vi "Manual Mode Update Vacuum.vi"(8 "error in":errorcluster, 10 "Vacuum Status":T1, 11 "Gantry in":refnum<class "Gantry Class.lvclass">) -> (0 "error out":errorcluster, 3 "Gantry out":refnum<class "Gantry Class.lvclass">)   [LabVIEW 2011]
uses:
  Shared Components/Gantry Class/Gantry Class.lvclass
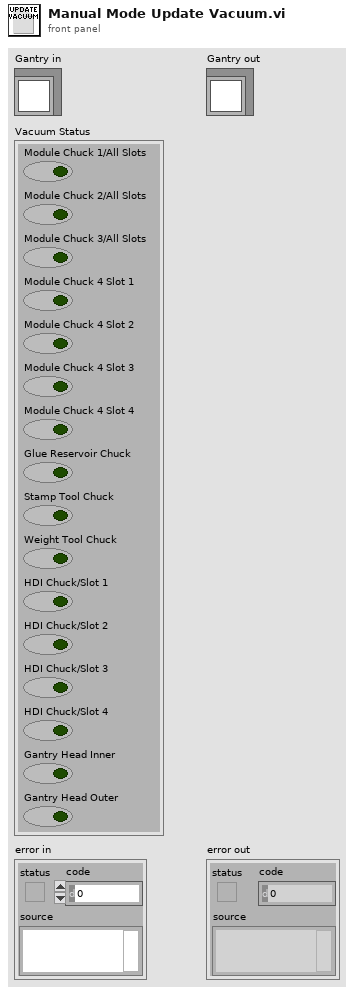
[diagram p1: front panel]
types:
  T1 = cluster{"Module Chuck 1/All Slots":bool, "Module Chuck 2/All Slots":bool, "Module Chuck 3/All Slots":bool, "Module Chuck 4 Slot 1":bool, "Module Chuck 4 Slot 2":bool, "Module Chuck 4 Slot 3":bool, "Module Chuck 4 Slot 4":bool, "Glue Reservoir Chuck":bool, "Stamp Tool Chuck":bool, "Weight Tool Chuck":bool, "HDI Chuck/Slot 1":bool, "HDI Chuck/Slot 2":bool, "HDI Chuck/Slot 3":bool, "HDI Chuck/Slot 4":bool, "Gantry Head Inner":bool, "Gantry Head Outer":bool}
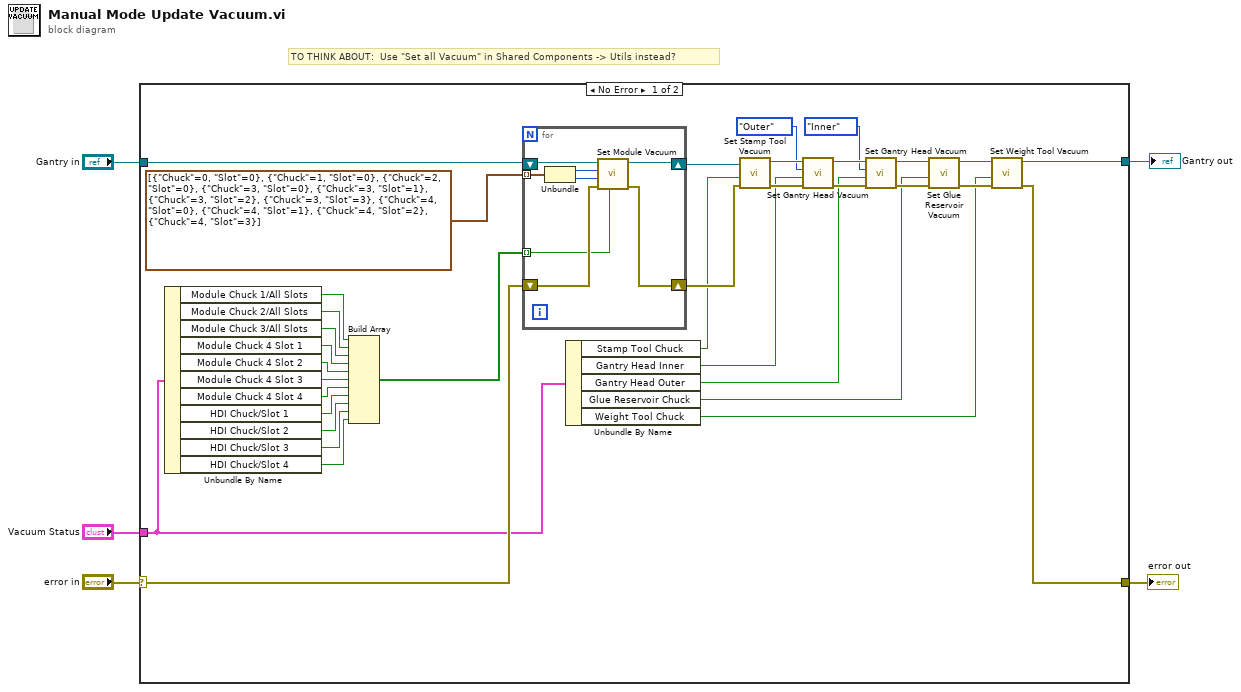
[diagram p0: block diagram]
diagram:
  # "TO THINK ABOUT:  Use \"Set all Vacuum\" in Shared Components -> Utils instead?"
  n1 = case shown="No Error" "error in" {
    selector: "error in" -> [w40 w49]
    tunnel: [w20 w49] -> w5
    tunnel: "Gantry in" -> [w28 w50]
    tunnel: "Vacuum Status" -> [w13 _]
    tunnel: [w22 w50] -> w1
    frame No Error {
      n2 = Unbundle By Name(w13) -> ("Module Chuck 1/All Slots"=w39:bool, "Module Chuck 2/All Slots"=w38:bool, "Module Chuck 3/All Slots"=w37:bool, "Module Chuck 4 Slot 1"=w36:bool, "Module Chuck 4 Slot 2"=w35:bool, "Module Chuck 4 Slot 3"=w34:bool, "Module Chuck 4 Slot 4"=w33:bool, "HDI Chuck/Slot 1"=w32:bool, "HDI Chuck/Slot 2"=w31:bool, "HDI Chuck/Slot 3"=w30:bool, "HDI Chuck/Slot 4"=w29:bool)
      n3 = Build Array(w39, w38, w37, w36, w35, w34, w33, w32, w31, w30, w29) -> (w27:bool[])
      n4 = for {
        shift-right: [w48] -> w21
        shift-left: w40 -> [w47]
        tunnel: w27 -> [w45] mode=indexing
        tunnel: cluster{"Chuck":i32, "Slot":i32}[] [{"Chuck"=0, "Slot"=0}, {"Chuck"=1, "Slot"=0}, {"Chuck"=2, "Slot"=0}, {"Chuck"=3, "Slot"=0}, {"Chuck"=3, "Slot"=1}, {"Chuck"=3, "Slot"=2}, {"Chuck"=3, "Slot"=3}, {"Chuck"=4, "Slot"=0}, {"Chuck"=4, "Slot"=1}, {"Chuck"=4, "Slot"=2}, {"Chuck"=4, "Slot"=3}] -> [w44] mode=indexing
        shift-right: [w41] -> w25
        shift-left: w28 -> [w46]
        n5 = Unbundle(w44) -> ("Chuck"=w43:i32, "Slot"=w42:i32)
        n6 = call-dynamic "Set Module Vacuum.vi"("On/Off"=w45, "error in"=w47, "Slot Number"=w42, "Chuck Number"=w43, "Gantry in"=w46) -> ("error out"=w48:errorcluster, "Gantry out"=w41:refnum<class "Gantry Class.lvclass">)  [unwired: 5 in]
      }
      n7 = Unbundle By Name(w13) -> ("Stamp Tool Chuck"=w12:bool, "Gantry Head Inner"=w11:bool, "Gantry Head Outer"=w10:bool, "Glue Reservoir Chuck"=w9:bool, "Weight Tool Chuck"=w8:bool)
      n8 = call-dynamic "Set Stamp Tool Vacuum.vi"("error in"=w21, "On/Off"=w12, "Gantry in"=w25) -> ("error out"=w19:errorcluster, "Gantry out"=w24:refnum<class "Gantry Class.lvclass">)  [unwired: 7 in]
      n9 = call-dynamic "Set Gantry Head Vacuum.vi"("error in (no error)"=w19, "On/Off"=w11, "Inner/Outer"=enum16{"Outer", "Inner"}."Outer", "Gantry Class in"=w24) -> ("error out"=w16:errorcluster, "Gantry Class out"=w17:refnum<class "Gantry Class.lvclass">)  [unwired: 6 in]
      n10 = call-dynamic "Set Gantry Head Vacuum.vi"("error in (no error)"=w16, "On/Off"=w10, "Inner/Outer"=enum16{"Outer", "Inner"}."Inner", "Gantry Class in"=w17) -> ("error out"=w14:errorcluster, "Gantry Class out"=w15:refnum<class "Gantry Class.lvclass">)  [unwired: 6 in]
      n11 = call-dynamic "Set Glue Reservoir Vacuum.vi"("error in (no error)"=w14, "On/Off"=w9, "Gantry Class in"=w15) -> ("error out"=w18:errorcluster, "Gantry Class out"=w23:refnum<class "Gantry Class.lvclass">)  [unwired: 7 in]
      n12 = call-dynamic "Set Weight Tool Vacuum.vi"("error in"=w18, "On/Off"=w8, "Gantry in"=w23) -> ("error out"=w20:errorcluster, "Gantry out"=w22:refnum<class "Gantry Class.lvclass">)  [unwired: 7 in]
    }
    frame Error {
    }
  }
  "Gantry out" <- w1
  "error out" <- w5
